vi "move template project.vi"(8 "error in":errorcluster, 10 "template path":path, 11 "CD name":string) -> (0 "error out":errorcluster, 3 "completed project":path)   [LabVIEW 2014, in "CD model script.lvlib"]
uses:
  CD model script.lvlib
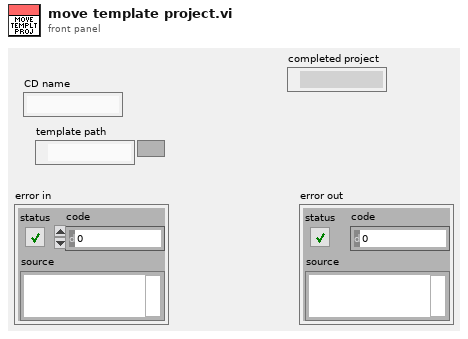
[diagram p1: front panel]
types:
  T1 = enum16{"open", "replace", "create", "open or create", "replace or create", "replace or create with confirmation"}
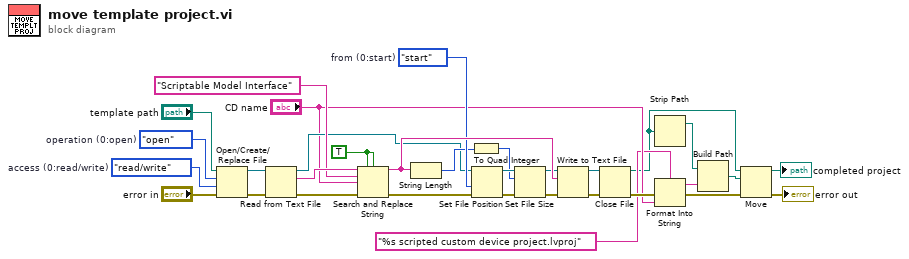
[diagram p0: block diagram]
diagram:
  w17 = enum16{"start", "end", "current"}."start"  # from (0:start)
  w24 = TRUE ("replace all? (F)")
  w28 = T1."open"  # operation (0:open)
  w29 = enum16{"read/write", "read-only", "write-only"}."read/write"  # access (0:read/write)
  n1 = Open/Create/Replace File(file path (use dialog)="template path", error in="error in", operation (0:open)=w28, access (0:read/write)=w29) -> (refnum out=w31:refnum<file>, error out=w30:errorcluster)  [unwired: 3 out]
  n2 = Read from Text File(file (use dialog)=w31, error in=w30) -> (refnum out=w14:refnum<file>, text=w27:string, error out=w26:errorcluster)  [unwired: 3 out]
  n3 = Search and Replace String(replace all?=w24, case sensitive?=w24, input string=w27, search string="Scriptable Model Interface", replace string="CD name", error in=w26) -> (result string=w32:string, error out=w13:errorcluster)  [unwired: 2 in, 2 out]
  n4 = String Length(string=w32) -> (length=w16:i32)
  n5 = To Quad Integer(1:w16) -> (0:w15:i64)
  n6 = Set File Position(refnum=w14, from (0:start)=w17, error in=w13) -> (refnum out=w18:refnum<file>, error out=w19:errorcluster)  [unwired: 1 out]
  n7 = Set File Size(4:w19, 6:w15, 7:w18) -> (0:w21:errorcluster, 3:w20:refnum<file>)
  n8 = Write to Text File(file (use dialog)=w20, text=w32, error in=w21) -> (refnum out=w23:refnum<file>, error out=w22:errorcluster)  [unwired: 2 out]
  n9 = Close File(refnum=w23, error in=w22) -> (path=w4:path, error out=w11:errorcluster)
  n10 = Strip Path(path=w4) -> (stripped path=w5:path)  [unwired: 1 out]
  n11 = Format Into String(format string="%s scripted custom device project.lvproj", error in=w11, "CD name") -> (resulting string=w2:string, error out=w9:errorcluster)  [unwired: 1 in]
  n12 = Build Path(base path=w5, name or relative path=w2) -> (appended path=w3:path)
  n13 = Move(source path=w4, error in=w9, 10:w3) -> (error out=→"error out":errorcluster, 3:→"completed project":path)  [unwired: 2 in, 1 out]
